vi "Disable Range Elements.vi"(10 "Use Default Limits":bool, 11 "Representation Enum":T1) -> (3 "Disabled?":T2(ring))   [LabVIEW 2018, in "Numeric Data Type.lvclass"]
uses:
  Numeric Data Type.lvclass
  Representation Enum.ctl
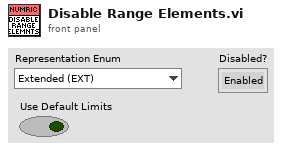
[diagram p1: front panel]
types:
  T1 = typedef "Numeric Data Type.lvclass/Representation Enum.ctl" = enum16{"Extended (EXT)", "Double (DBL)", "Single (SGL)", "Fixed-Point (FXP)", "Quad Integer (I64)", "Long Integer (I32)", "Word Integer (I16)", "Byte Integer (I8)", "Unsigned Quad (U64)", "Unsigned Long (U32)", "Unsigned Word (U16)", "Unsigned Byte (U8)", "Complex Extended (CXT)", "Complex Double (CDB)", "Complex Single (CSG)"}
  T2 = enum8{"Enabled", "Disabled", "Disabled and Grayed Out"}
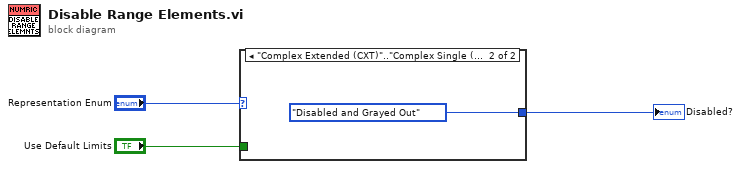
[diagram p0: block diagram]
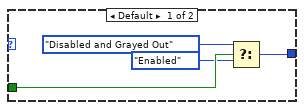
[diagram p2: hidden frame]
diagram:
  n1 = case shown="\"Complex Extended (CXT)\"..\"Complex Single (CSG)\"" "Representation Enum" {
    tunnel: [w4 T2."Disabled and Grayed Out" ("Disabled")] -> w2
    tunnel: "Use Default Limits" -> [w7 _]
    frame Default {
      n2 = Select(t=T2."Disabled and Grayed Out" ("Disabled"), s=w7, f=T2."Enabled" ("Disabled")) -> (s? t:f=w4:T2)
    }
    frame "Complex Extended (CXT)".."Complex Single (CSG)" {
    }
  }
  "Disabled?" <- w2
